vi "GVHA Gas Viscosity of Humid Air (Kg to m to s).vi"(1 "Gas Presure":dbl[unit]=80000.0 min=80000.0 max=120000.0, 2 "Tceg":dbl[unit], 3 "RH":dbl) -> (0 "Gas Viscosity Of  Humid Air":dbl[unit])   [LabVIEW 2018]
panel:
  out "Temprature Of Input Air\nKelvin Degree":dbl[unit](slide) scale=273.0..373.0
  out "Temprature Of Input Air\nCentigrade Degree":dbl[unit](slide) scale=0.0..100.0
  out "Humidity of Input Air":dbl(knob) scale=0.0..100.0
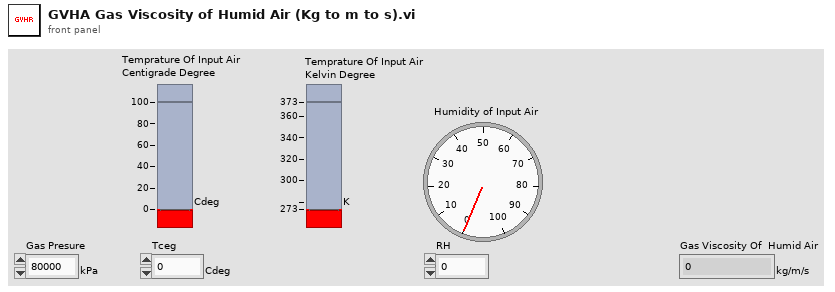
[diagram p1: front panel]
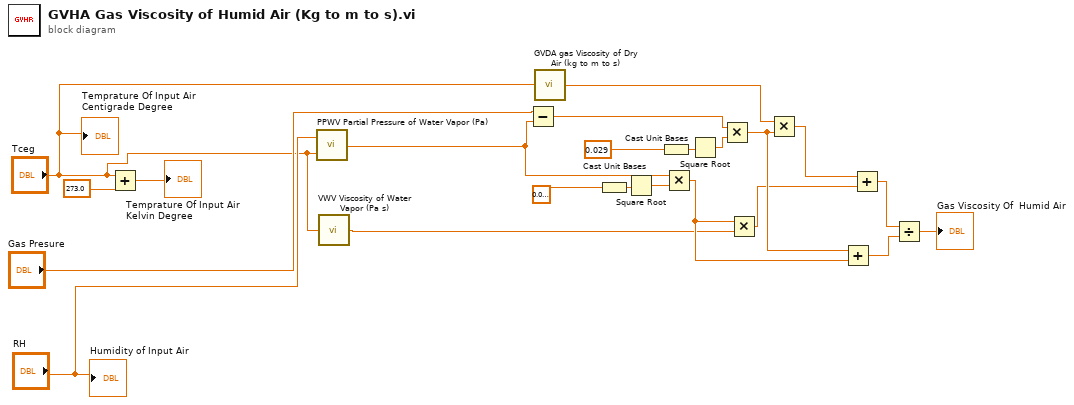
[diagram p0: block diagram]
diagram:
  n1 = Add(x="Tceg", y=dbl[unit] 273.0) -> (x+y=→"Temprature Of Input Air\nKelvin Degree":dbl[unit])
  n2 = call "PPWV Partial Pressure of Water Vapor (Pa).vi"("Tceg"="Tceg", "RH"="RH") -> ("PPWV"=w8:dbl[unit])
  n3 = call "VWV Viscosity of Water Vapor (Pa s).vi"("Pure Water Temprature"="Tceg") -> ("Visocity of  Water Vapor"=w1:dbl[unit])
  n4 = Subtract(x="Gas Presure", y=w8) -> (x-y=w12:dbl[unit])
  n5 = call "GVDA gas Viscosity of Dry Air (kg to m to s).vi"("Tceg\nGas Temperature"="Tceg") -> ("Gas Viscosity\nof Dry Air"=w10:dbl[unit])
  n6 = Cast Unit Bases(0:dbl[unit] 0.018000000000000002 ("y")) -> (2:w7:dbl)  [unwired: 1 in]
  n7 = Square Root(x=w7) -> (sqrt(x)=w6:dbl)
  n8 = Cast Unit Bases(0:dbl[unit] 0.029 ("y")) -> (2:w17:dbl)  [unwired: 1 in]
  n9 = Multiply(x=w8, y=w6) -> (x*y=w2:dbl[unit])
  n10 = Square Root(x=w17) -> (sqrt(x)=w11:dbl)
  n11 = Multiply(x=w12, y=w11) -> (x*y=w9:dbl[unit])
  n12 = Multiply(x=w2, y=w1) -> (x*y=w4:dbl[unit])
  n13 = Multiply(x=w10, y=w9) -> (x*y=w18:dbl[unit])
  n14 = Add(x=w9, y=w2) -> (x+y=w19:dbl[unit])
  n15 = Add(x=w18, y=w4) -> (x+y=w20:dbl[unit])
  n16 = Divide(x=w20, y=w19) -> (x/y=→"Gas Viscosity Of  Humid Air":dbl[unit])
  "Humidity of Input Air" <- "RH"
  "Temprature Of Input Air\nCentigrade Degree" <- "Tceg"
